vi "g1.vi"(1 "stop":bool, 2 "Sygna³":T1(ring), 3 "Amplituda":dbl(knob) scale=0.0..10.0, 4 "Czêstotliwoœæ":dbl(knob) scale=0.0..10.0) -> (0 "Charakterystyka":waveform(dbl)(graph))   [LabVIEW 2020]
uses:
  <vilib>/measure/NI_MABase.lvlib
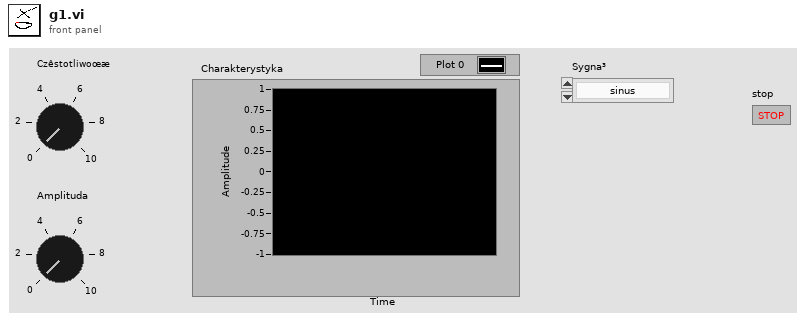
[diagram p1: front panel]
types:
  T1 = enum16{"sinus\n", "square\n", "triangle\n", "sawtooth\n"}
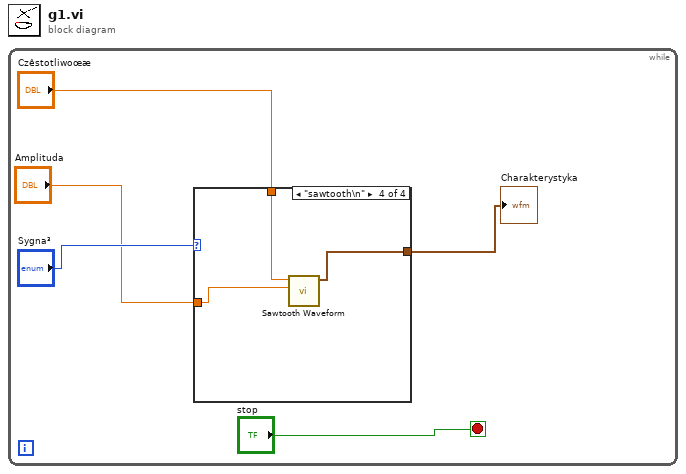
[diagram p0: block diagram]
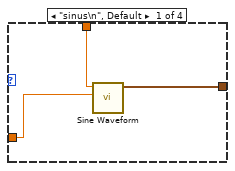
[diagram p2: hidden frame]
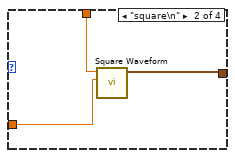
[diagram p3: hidden frame]
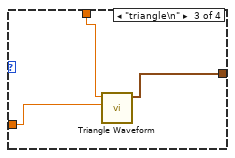
[diagram p4: hidden frame]
diagram:
  n1 = while {
    stop <- "stop" stop-if-true
    n2 = case shown="\"sawtooth\\n\"" "Sygna³" {
      tunnel: "Amplituda" -> [w8 w11 w14 w16]
      tunnel: "Czêstotliwoœæ" -> [w7 w10 w13 w17]
      tunnel: [w6 w9 w12 w15] -> w1
      frame "sinus\n", Default {
        n3 = call <vilib>:"Sine Waveform.vi"("amplitude"=w8, "frequency"=w7) -> ("signal out"=w6:waveform(dbl))  [unwired: 8 in, 1 out]
      }
      frame "square\n" {
        n4 = call <vilib>:"Square Waveform.vi"("amplitude"=w11, "frequency"=w10) -> ("signal out"=w9:waveform(dbl))  [unwired: 8 in, 1 out]
      }
      frame "triangle\n" {
        n5 = call <vilib>:"Triangle Waveform.vi"("amplitude"=w14, "frequency"=w13) -> ("signal out"=w12:waveform(dbl))  [unwired: 8 in, 1 out]
      }
      frame "sawtooth\n" {
        n6 = call <vilib>:"Sawtooth Waveform.vi"("amplitude"=w16, "frequency"=w17) -> ("signal out"=w15:waveform(dbl))  [unwired: 8 in, 1 out]
      }
    }
    "Charakterystyka" <- w1
  }
